vi "Joystick2RobotMotorCommands.vi"(9 "Joystick R":dbl, 10 "Joystick Y":dbl, 11 "Joystick X":dbl) -> (3 "Robot Motion Commands":T1)   [LabVIEW 2018]
uses:
  Robot Pivot Motion Commands.ctl
  Pivot Motor Commands.ctl
  Robot Drive Mode.ctl
panel:
  out "D":dbl
  out "C":dbl
  out "B":dbl
  out "A":dbl
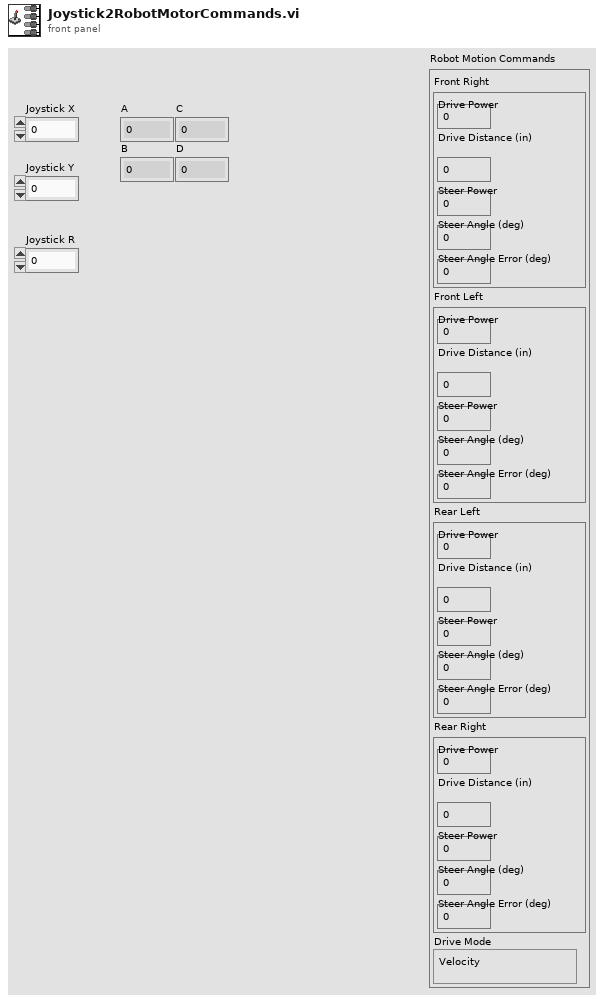
[diagram p1: front panel]
types:
  T1 = typedef "Robot Pivot Motion Commands.ctl" = cluster{"Front Right":T2, "Front Left":T2, "Rear Left":T2, "Rear Right":T2, "Drive Mode":T3}
  T2 = typedef "Pivot Motor Commands.ctl" = cluster{"Drive Power":dbl, "Drive Distance (in)":dbl, "Steer Power":dbl, "Steer Angle (deg)":dbl, "Steer Angle Error (deg)":dbl}
  T3 = typedef "Robot Drive Mode.ctl" = enum16{"Velocity", "Distance"}
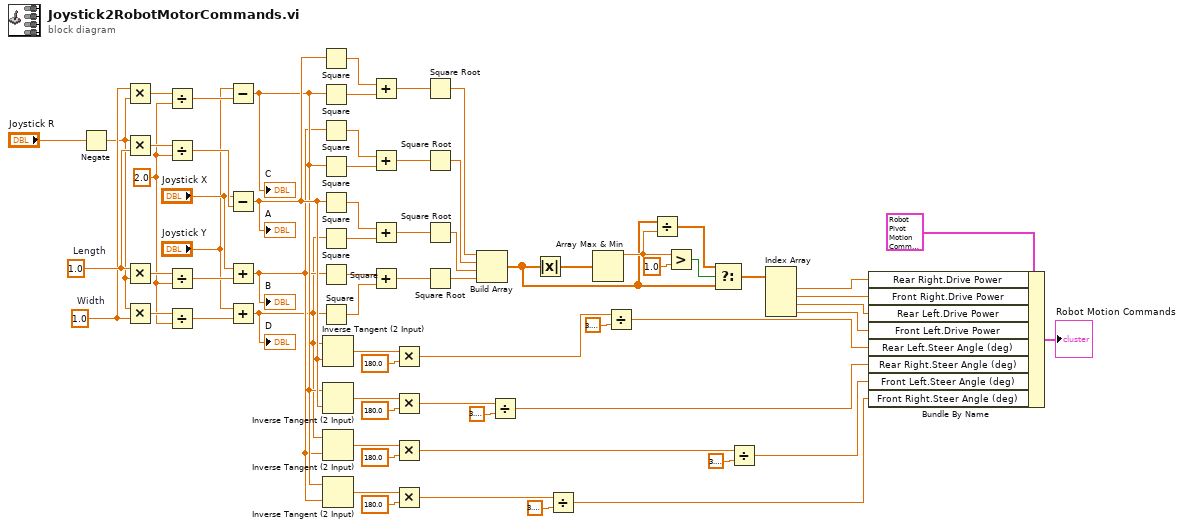
[diagram p0: block diagram]
diagram:
  w27 = 2.0
  w28 = 1.0  # Width
  w65 = 1.0  # Length
  n1 = Negate(x="Joystick R") -> (-x=w22:dbl)
  n2 = Multiply(x=w28, y=w22) -> (x*y=w62:dbl)
  n3 = Multiply(x=w22, y=w65) -> (x*y=w68:dbl)
  n4 = Multiply(x=w65, y=w22) -> (x*y=w64:dbl)
  n5 = Multiply(x=w22, y=w28) -> (x*y=w59:dbl)
  n6 = Divide(x=w62, y=w27) -> (x/y=w61:dbl)
  n7 = Divide(x=w68, y=w27) -> (x/y=w67:dbl)
  n8 = Divide(x=w64, y=w27) -> (x/y=w63:dbl)
  n9 = Divide(x=w59, y=w27) -> (x/y=w58:dbl)
  n10 = Subtract(x="Joystick Y", y=w61) -> (x-y=w25:dbl)
  "C" <- w25
  n11 = Subtract(x="Joystick X", y=w67) -> (x-y=w26:dbl)
  "A" <- w26
  n12 = Add(x="Joystick X", y=w63) -> (x+y=w24:dbl)
  "B" <- w24
  n13 = Add(x="Joystick Y", y=w58) -> (x+y=w23:dbl)
  "D" <- w23
  n14 = Square(x=w26) -> (x^2=w32:dbl)
  n15 = Square(x=w25) -> (x^2=w31:dbl)
  n16 = Square(x=w24) -> (x^2=w53:dbl)
  n17 = Square(x=w25) -> (x^2=w52:dbl)
  n18 = Square(x=w26) -> (x^2=w39:dbl)
  n19 = Square(x=w23) -> (x^2=w38:dbl)
  n20 = Square(x=w24) -> (x^2=w46:dbl)
  n21 = Square(x=w23) -> (x^2=w45:dbl)
  n22 = Inverse Tangent (2 Input)(1:w26, 2:w23) -> (0:w43:dbl)
  n23 = Inverse Tangent (2 Input)(1:w26, 2:w25) -> (0:w36:dbl)
  n24 = Inverse Tangent (2 Input)(1:w24, 2:w23) -> (0:w50:dbl)
  n25 = Inverse Tangent (2 Input)(1:w24, 2:w25) -> (0:w57:dbl)
  n26 = Add(x=w32, y=w31) -> (x+y=w30:dbl)
  n27 = Add(x=w53, y=w52) -> (x+y=w51:dbl)
  n28 = Add(x=w39, y=w38) -> (x+y=w37:dbl)
  n29 = Add(x=w46, y=w45) -> (x+y=w44:dbl)
  n30 = Multiply(x=w43, y=180.0) -> (x*y=w40:dbl)
  n31 = Multiply(x=w36, y=180.0) -> (x*y=w34:dbl)
  n32 = Multiply(x=w50, y=180.0) -> (x*y=w47:dbl)
  n33 = Multiply(x=w57, y=180.0) -> (x*y=w54:dbl)
  n34 = Square Root(x=w30) -> (sqrt(x)=w21:dbl)
  n35 = Square Root(x=w51) -> (sqrt(x)=w20:dbl)
  n36 = Square Root(x=w37) -> (sqrt(x)=w19:dbl)
  n37 = Square Root(x=w44) -> (sqrt(x)=w18:dbl)
  n38 = Build Array(w21, w20, w19, w18) -> (w12:dbl[])
  n39 = Divide(x=w34, y=3.141592653589793) -> (x/y=w5:dbl)
  n40 = Absolute Value(x=w12) -> (abs(x)=w17:dbl[])
  n41 = Divide(x=w54, y=3.141592653589793) -> (x/y=w3:dbl)
  n42 = Array Max & Min(array=w17) -> (max value=w14:dbl)  [unwired: 3 out]
  n43 = Divide(x=w40, y=3.141592653589793) -> (x/y=w6:dbl)
  n44 = Divide(x=w12, y=w14) -> (x/y=w13:dbl[])
  n45 = Greater?(x=w14, y=1.0) -> (0:w15:bool)
  n46 = Select(t=w13, s=w15, f=w12) -> (s? t:f=w11:dbl[])
  n47 = Divide(x=w47, y=3.141592653589793) -> (x/y=w4:dbl)
  n48 = Index Array(array=w11) -> (element #1=w10:dbl, element #2=w9:dbl, element #3=w8:dbl, element #4=w7:dbl)  [unwired: 4 in]
  n49 = Bundle By Name(cluster=T1 {"Front Right"={"Drive Power"=0.0, "Drive Distance (in)"=0.0, "Steer Power"=0.0, "Steer Angle (deg)"=0.0, "Steer Angle Error (deg)"=0.0}, "Front Left"={"Drive Power"=0.0, "Drive Distance (in)"=0.0, "Steer Power"=0.0, "Steer Angle (deg)"=0.0, "Steer Angle Error (deg)"=0.0}, "Rear Left"={"Drive Power"=0.0, "Drive Distance (in)"=0.0, "Steer Power"=0.0, "Steer Angle (deg)"=0.0, "Steer Angle Error (deg)"=0.0}, "Rear Right"={"Drive Power"=0.0, "Drive Distance (in)"=0.0, "Steer Power"=0.0, "Steer Angle (deg)"=0.0, "Steer Angle Error (deg)"=0.0}, "Drive Mode"=enum."Velocity"} ("Robot Motion Commands 2"), "Rear Right.Drive Power"=w10, "Front Right.Drive Power"=w9, "Rear Left.Drive Power"=w8, "Front Left.Drive Power"=w7, "Rear Left.Steer Angle (deg)"=w6, "Rear Right.Steer Angle (deg)"=w5, "Front Left.Steer Angle (deg)"=w4, "Front Right.Steer Angle (deg)"=w3) -> (→"Robot Motion Commands":T1)
